vi "ESNsub_RandomMatrix.vi"(9 "Range (1)":dbl=1.0, 10 "Column":i32, 11 "Row":i32) -> (3 "Matrix":dbl[][](array[numeric]))   [LabVIEW 2017]
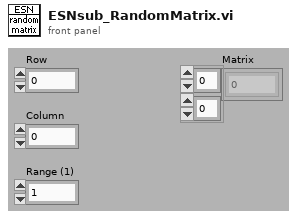
[diagram p1: front panel]
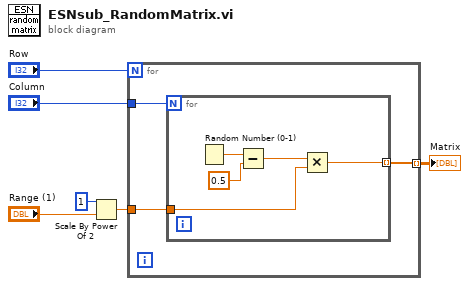
[diagram p0: block diagram]
diagram:
  n1 = Scale By Power Of 2(n=1, x="Range (1)") -> (x*2^n=w1:dbl)
  n2 = for {
    N: "Row" -> [_]
    tunnel: "Column" -> [w9]
    tunnel: [w8] -> w4 mode=indexing
    tunnel: w1 -> [w7]
    n3 = for {
      N: w9 -> [_]
      tunnel: [w11] -> w8 mode=indexing
      tunnel: w7 -> [w10]
      n4 = Random Number (0-1)() -> (number: 0 to 1=w14:dbl)
      n5 = Subtract(x=w14, y=0.5) -> (x-y=w12:dbl)
      n6 = Multiply(x=w12, y=w10) -> (x*y=w11:dbl)
    }
  }
  "Matrix" <- w4
